vi "DAQmx Set CJC Parameters (sub).vi"(0 "task in":refnum<k21>, 5 "thermocouple channel":string, 7 "cjc source":i32(ring)=10200 items=["Built-In"=10200, "Constant Value"=10116, "Channel"=10113], 9 "cjc channel":string, 11 "error in":errorcluster) -> (4 "task out":refnum<k21>, 15 "error out":errorcluster)   [LabVIEW 2013]
uses:
  nilvaiu.dll
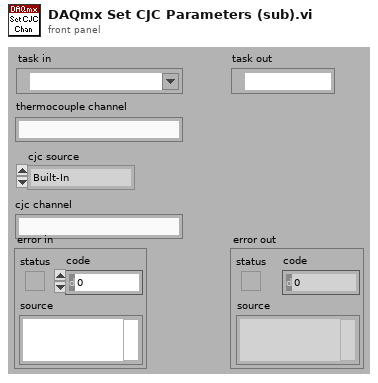
[diagram p1: front panel]
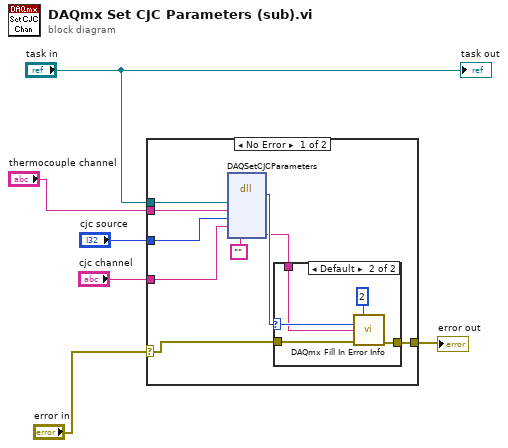
[diagram p0: block diagram]
diagram:
  n1 = case shown="No Error" "error in" {
    selector: "error in" -> [w8 w22]
    tunnel: "task in" -> [w15 _]
    tunnel: "thermocouple channel" -> [w14 _]
    tunnel: "cjc source" -> [w13 _]
    tunnel: "cjc channel" -> [w12 _]
    tunnel: [w7 w22] -> w2
    frame No Error {
      n2 = dll-call lib="nilvaiu.*" fn="DAQSetCJCParameters"("taskID"=w15, "activeChannel"=w14, "cjcType"=w13, "cjcChannel"=w12, "extendedErrorInfo"="") -> (w10:i32, "extendedErrorInfo"=w9:string)  [unwired: 6 in, 3 out]
      n3 = case shown="Default" w10 {
        selector: w10 -> [_ w20]
        tunnel: [w16 w21] -> w7
        tunnel: w9 -> [_ w19]
        tunnel: w8 -> [w16 w18]
        frame 0 {
        }
        frame Default {
          n4 = call "DAQmx Fill In Error Info.vi"("depth"=2, "status code"=w20, "extended error info"=w19, "error in"=w18) -> ("error out"=w21:errorcluster)  [unwired: 1 in, 10 out]
        }
      }
    }
    frame Error {
    }
  }
  "error out" <- w2
  "task out" <- "task in"
